vi "DrawAxesOnImageFromClusters (SubVI).vi"(0 "Image Refnum in":T1, 1 "X Value":dbl, 2 "Y Value":dbl, 5 "X Minimum":dbl, 7 "X Maximum":dbl, 11 "error in (no error)":errorcluster, 12 "Y Minimum":dbl, 13 "Y Maximum":dbl, 14 "Axes colour":u32(colorbox)=16711680) -> (4 "Image Refnum out":T1, 15 "error out":errorcluster)   [LabVIEW 2016]
uses:
  <vilib>/vision/Image Controls.llb/IMAQ Image.ctl
panel:
  # "This SubVI draws axes centered on (X Value, Y Value) in image coordinate units\non the supplied image"
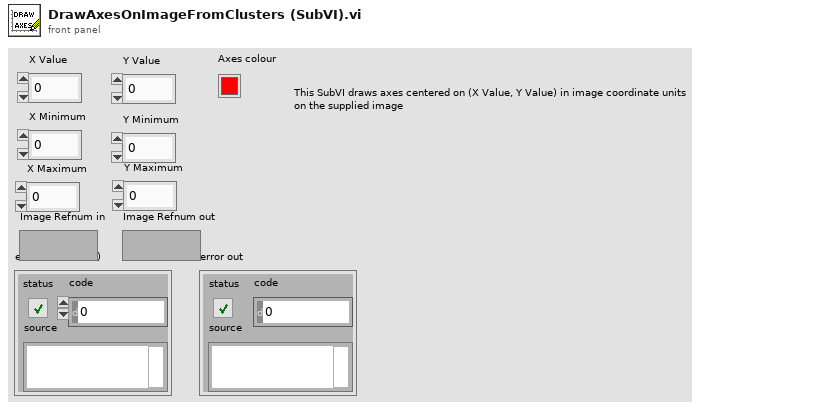
[diagram p1: front panel]
types:
  T1 = typedef "IMAQ Image.ctl" = refnum<image>
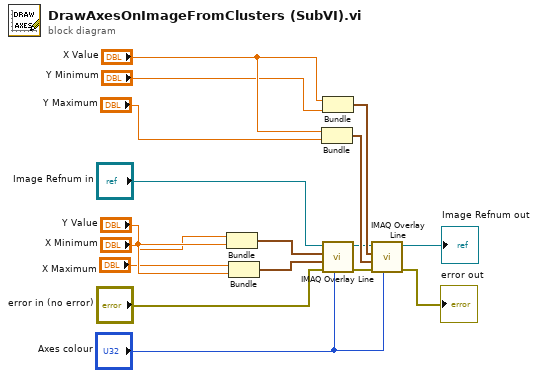
[diagram p0: block diagram]
diagram:
  n1 = Bundle("X Minimum"="X Minimum", "Y Value"="Y Value") -> (w16:cluster{"X Minimum":dbl, "Y Value":dbl})  [unwired: 1 in]
  n2 = Bundle("X Maximum"="X Maximum", "Y Value"="Y Value") -> (w15:cluster{"X Maximum":dbl, "Y Value":dbl})  [unwired: 1 in]
  n3 = Bundle("X Value"="X Value", "Y Maximum"="Y Maximum") -> (w13:cluster{"X Value ":dbl, "Y Maximum":dbl})  [unwired: 1 in]
  n4 = Bundle("X Value"="X Value", "Y Minimum"="Y Minimum") -> (w14:cluster{"X Value ":dbl, "Y Minimum":dbl})  [unwired: 1 in]
  n5 = call "IMAQ Overlay Line"("Color"="Axes colour", "error in (no error)"="error in (no error)", "End Point"=w15, "Start Point"=w16, "Image"="Image Refnum in") -> ("error out"=w9:errorcluster, "Image Out"=w12:T1)  [unwired: 5 in]
  n6 = call "IMAQ Overlay Line"("Color"="Axes colour", "error in (no error)"=w9, "End Point"=w13, "Start Point"=w14, "Image"=w12) -> ("error out"=→"error out":errorcluster, "Image Out"=→"Image Refnum out":T1)  [unwired: 5 in]
